vi "Get Pin Map Path.vi"(8 "error in":errorcluster, 10 "Sequence Context In":refnum<k7>, 11 "Pin Map Name":string) -> (0 "error out":errorcluster, 3 "Pin Map Path":string)   [LabVIEW 2020, in "NIDCPowerSourceDCVoltage.lvlib"]
uses:
  NIDCPowerSourceDCVoltage.lvlib
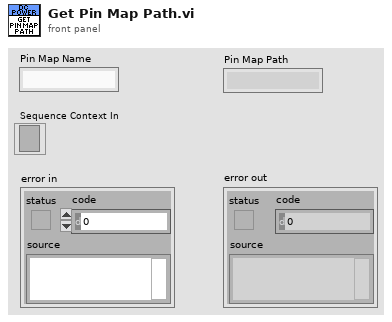
[diagram p1: front panel]
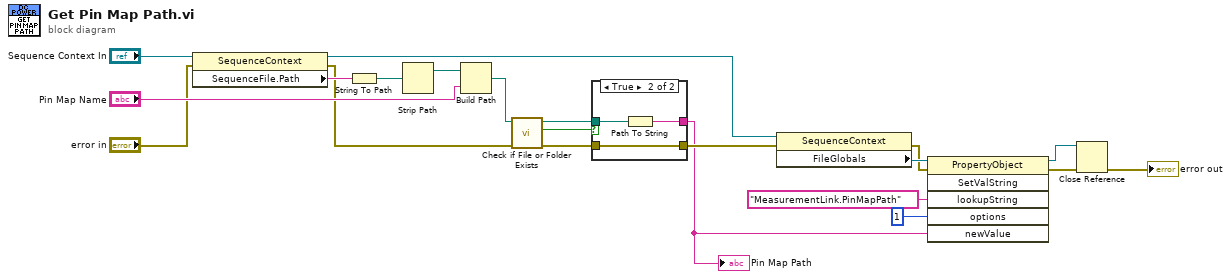
[diagram p0: block diagram]
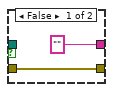
[diagram p2: hidden frame]
diagram:
  n1 = property class="SequenceContext"(reference="Sequence Context In", error in="error in") -> (reference out=w7:refnum<k7>, error out=w11:errorcluster, "SequenceFile.Path"=w17:string)
  n2 = String To Path(string=w17) -> (path=w18:path)
  n3 = Strip Path(path=w18) -> (stripped path=w20:path)  [unwired: 1 out]
  n4 = Build Path(base path=w20, name or relative path="Pin Map Name") -> (appended path=w19:path)
  n5 = call <vilib>:"Check if File or Folder Exists.vi"("error in (no error)"=w11, "path"=w19) -> ("error out"=w13:errorcluster, "file or folder exists?"=w15:bool, "dup path"=w14:path)  [unwired: 7 in]
  n6 = case shown="True" w15 {
    tunnel: w14 -> [_ w26]
    tunnel: ["" w25] -> w4
    tunnel: w13 -> [w22 w24]
    tunnel: [w22 w24] -> w6
    frame False {
    }
    frame True {
      n7 = Path To String(path=w26) -> (string=w25:string)
    }
  }
  "Pin Map Path" <- w4
  n8 = property class="SequenceContext"(reference=w7, error in=w6) -> (error out=w5:errorcluster, "FileGlobals"=w10:refnum<k7>)  [unwired: 1 out]
  n9 = invoke class="PropertyObject" method="SetValString"(reference=w10, error in=w5, "lookupString"="MeasurementLink.PinMapPath", "options"=1, "newValue"=w4) -> (reference out=w2:refnum<k7>, error out=w3:errorcluster)  [unwired: 1 in, 4 out]
  n10 = Close Reference(reference=w2, error in (no error)=w3) -> (error out=→"error out":errorcluster)
